vi "Error_log.vi"(8 "error in (no error)":errorcluster, 11 "Step":string) -> (0 "error out":errorcluster, 2 "source":string, 3 "code":i32)   [LabVIEW 2014, in "Driver_interaction.lvlib" / "_Driver_interaction.lvclass"]
uses:
  _Driver_interaction.lvclass
  Deploy/Utilities/Miscelanous.lvlibp/Controls/Configuration_file.ctl
  <vilib>/Utility/file.llb/Write To Spreadsheet File (string).vi
  Deploy/Utilities/Miscelanous.lvlibp
panel:
  out "date/time string":string
  out "appended path":path
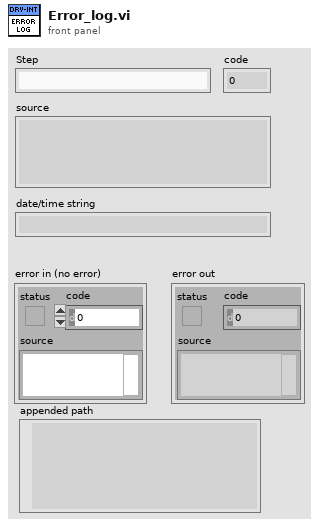
[diagram p1: front panel]
types:
  T1 = typedef "Miscelanous.lvlibp/Configuration_file.ctl" = enum16{"Station_settings", "Instrument_config", "Test_config", "Error_log", "Vision_maintenance", "Services", "Mapping_signals", "Failures"}
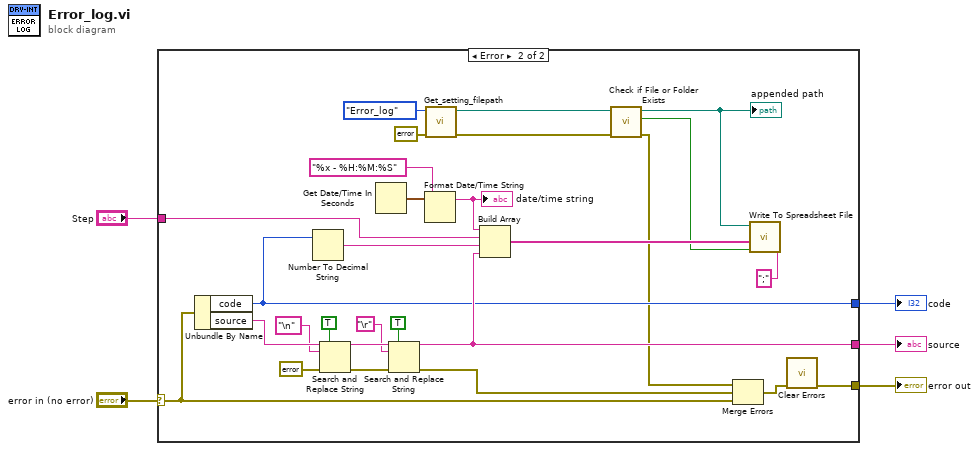
[diagram p0: block diagram]
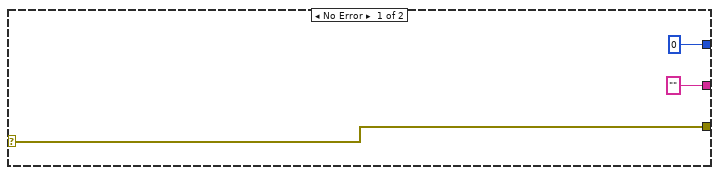
[diagram p2: hidden frame]
diagram:
  n1 = case shown="Error" "error in (no error)" {
    selector: "error in (no error)" -> [w8 w21]
    tunnel: [w8 w19] -> w3
    tunnel: "Step" -> [_ w27]
    tunnel: ["" ("result string") w29] -> w2
    tunnel: [0 ("code") w18] -> w1
    frame No Error {
    }
    frame Error {
      n2 = Unbundle By Name(w21) -> ("code"=w18:i32, "source"=w36:string)
      n3 = Number To Decimal String(number=w18) -> (decimal integer string=w28:string)  [unwired: 1 in]
      n4 = Search and Replace String(replace all?=TRUE ("replace all? (F)"), input string=w36, search string="\n", error in=errorcluster {"status"=FALSE, "code"=0, "source"=""} ("error in (no error)")) -> (result string=w34:string, error out=w35:errorcluster)  [unwired: 4 in, 2 out]
      n5 = Get Date/Time In Seconds() -> (seconds since 1Jan1904=w26:timestamp)
      n6 = Search and Replace String(replace all?=TRUE ("replace all? (F)"), input string=w34, search string="\r", error in=w35) -> (result string=w29:string, error out=w22:errorcluster)  [unwired: 4 in, 2 out]
      n7 = Format Date/Time String(time format string (%c)="%x - %H:%M:%S", seconds (now)=w26) -> (date/time string=w17:string)  [unwired: 1 in]
      "date/time string" <- w17
      n8 = call "Get_setting_filepath.vi"("error in (no error)"=errorcluster {"status"=FALSE, "code"=0, "source"=""}, "Configuration file"=Configuration_file."Error_log") -> ("error out"=w14:errorcluster, "Settings filepath"=w12:path)  [unwired: 7 in, 1 out]
      n9 = Build Array(w17, w27, w28, w29) -> (w24:string[])
      n10 = call <vilib>:"Check if File or Folder Exists.vi"("error in (no error)"=w14, "path"=w12) -> ("error out"=w13:errorcluster, "file or folder exists?"=w15:bool, "dup path"=w11:path)  [unwired: 7 in]
      "appended path" <- w11
      n11 = Merge Errors(w13, w22, w21) -> (w20:errorcluster)
      n12 = call-poly <vilib>:"Write To Spreadsheet File.vi"("delimiter (\\t)"=";" ("delimiter (\\t)"), "append to file? (new file:F)"=w15, "1D data"=w24, "file path (dialog if empty)"=w11) -> ()  [unwired: 4 in, 1 out]
      n13 = call <vilib>:"Clear Errors.vi"("error in (no error)"=w20) -> ("error out"=w19:errorcluster)  [unwired: 5 in, 1 out]
    }
  }
  "error out" <- w3
  "code" <- w1
  "source" <- w2
